vi "Shooter Speed Control.vi"(2 "Use Speed Control":bool=TRUE, 3 "Desired\nShooter\nSpeed":dbl) -> (1 "up to speed":bool)   [LabVIEW 2013]
panel:
  in  "counts/rev":dbl=240.0
  out "Wheel Speed R/sec":dbl=2.0076839341392278e-147 format="%#_4g"
  out "Count":i32=1335982
  in  "Reset Counter":bool
  in  "Speed avg. #":dbl=6.0
  in  "Gain":dbl=0.2
  in  "Allowable\nSpeed Error":dbl=2.0
  in  "Bias":dbl=99.0
  out "speed error":cluster{dbl, dbl}(graph)={-2.4092207209670736e-147, 0.017}
  # ".2"
  # "6"
  # "99"
  # "calibrate for \n50 rps with loop\ndisabled"
  # "240/360 depending\non which encoder\n\n81 on RPC test setup"
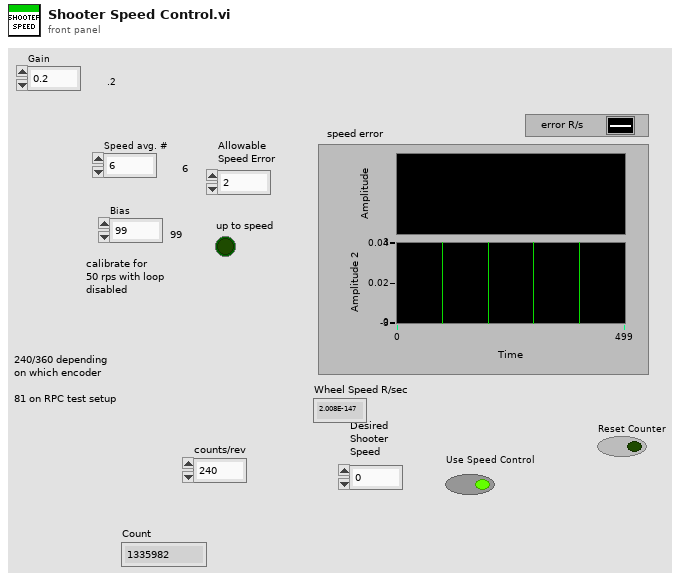
[diagram p1: front panel]
types:
  T1 = typedef "WPI_CounterDevRef.ctl" = cluster{"DevStatus":errorcluster, "CntIndex":T2}
  T2 = typedef "FPGA_CounterCtrSystemIndex.ctl" = enum8{"Ctr 0", "Ctr 1", "Ctr 2", "Ctr 3", "Ctr 4", "Ctr 5", "Ctr 6", "Ctr 7", "Invalid"}
  T3 = typedef "WPI_MotorControlDeviceRef.ctl" = cluster{"DeviceStatus":errorcluster, "Type":enum16{"PWM", "CAN"}, "PWM":cluster{"Digital Module":T4, "PWM Channel":T5, "DeadBand":T6}, "CAN":cluster{"Device Number":u8, "Control Mode":T7, "Semaphore":T8, "Max Vout":dbl}, "Invert":bool, "TransformRef":T9, "InvTransformRef":T9}
  T4 = typedef "FPGA_TypedefDigitalModule.ctl" = enum16{"Digital Module 1", "Digital Module 2"}
  T5 = typedef "FPGA_DIOPWMChannel.ctl" = enum8{"PWM 1", "PWM 2", "PWM 3", "PWM 4", "PWM 5", "PWM 6", "PWM 7", "PWM 8", "PWM 9", "PWM 10", "Invalid"}
  T6 = typedef "WPI_PWMDeadband.ctl" = cluster{"Name":string, "maxPositivePwm":i32, "minPositivePwm":i32, "centerPwm":i32, "maxNegativePwm":i32, "minNegativePwm":i32, "angularRange":u16}
  T7 = typedef "WPI_CANJaguar_ControlMode.ctl" = enum8{"Percent VBus", "Current", "Speed", "Position", "Voltage"}
  T8 = typedef "Semaphore RefNum" = refnum<k1>
  T9 = typedef "WPI_PWMTransform_ConPane.ctl" = refnum<vi>
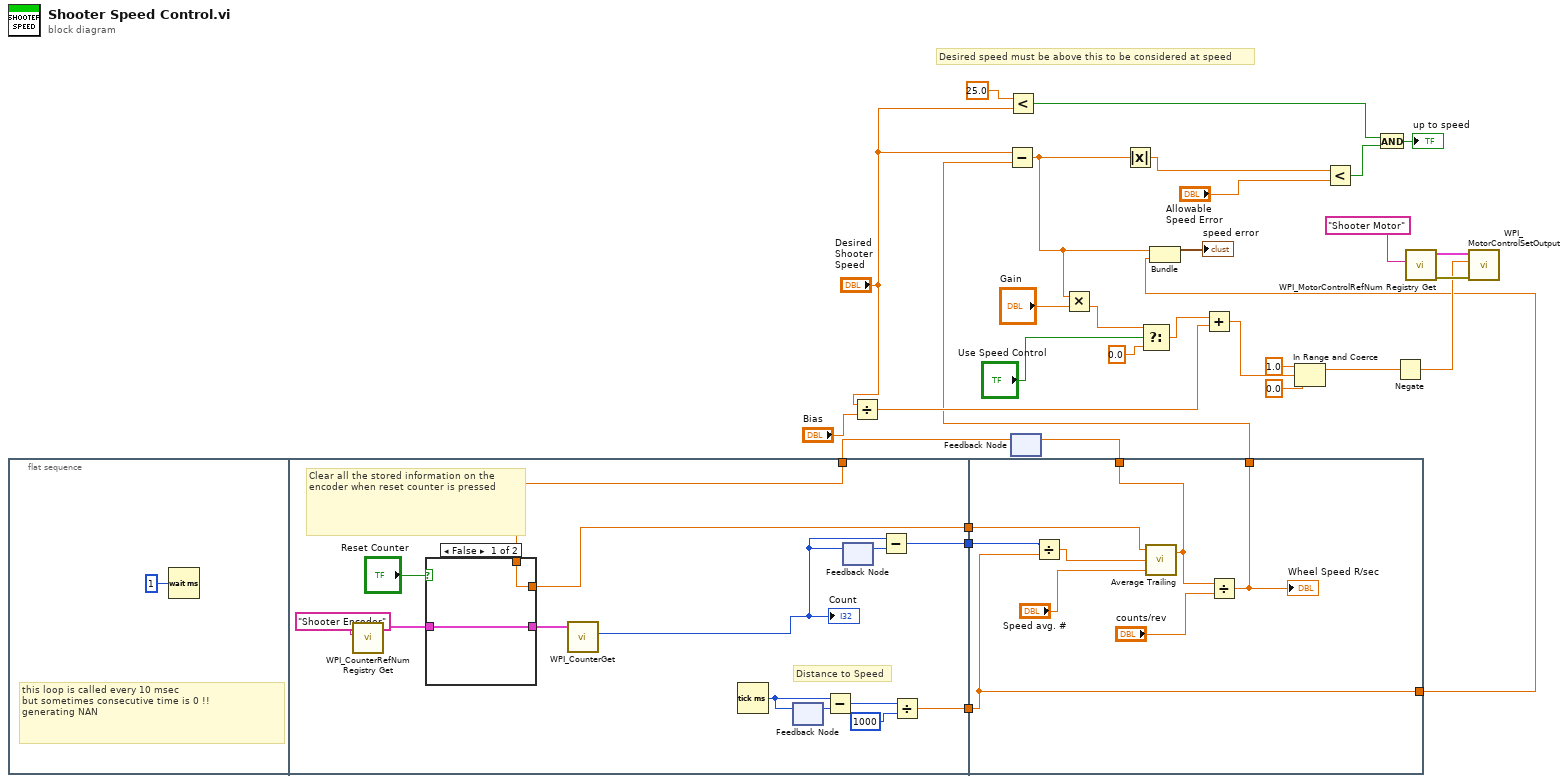
[diagram p0: block diagram]
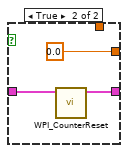
[diagram p2: hidden frame]
diagram:
  # "Desired speed must be above this to be considered at speed"
  n1 = flat-sequence {
    tunnel: [w36] -> w9
    tunnel: [w35] -> w8
    tunnel: [w34] -> w7
    tunnel: w1 -> [w33]
    tunnel: w9 -> [w56]
    tunnel: w8 -> [w54]
    tunnel: w7 -> [w55]
    tunnel: [w54] -> w6
    tunnel: [w53] -> w5
    tunnel: [w52] -> w2
    frame #0 {
      # "this loop is called every 10 msec\nbut sometimes consecutive time is 0 !!\ngenerating NAN"
      n2 = Wait (ms)(milliseconds to wait=u32 1) -> ()  [unwired: 1 out]
    }
    frame #1 {
      # "Distance to Speed"
      # "Clear all the stored information on the encoder when reset counter is pressed"
      n3 = call <vilib>:"WPI_CounterRefNum Registry Get.vi"("refnum name"="Shooter Encoder") -> ("CounterDevRef"=w41:T1)  [unwired: 9 in, 1 out]
      n4 = case shown="False" "Reset Counter" {
        tunnel: w41 -> [w48 w50]
        tunnel: [w48 w49] -> w38
        tunnel: w33 -> [w47 _]
        tunnel: [w47 0.0 ("Output")] -> w34
        frame False {
        }
        frame True {
          n5 = call <vilib>:"WPI_CounterReset.vi"("CounterDevRef in"=w50) -> ("CounterDevRef out"=w49:T1)  [unwired: 9 in, 1 out]
        }
      }
      n6 = call <vilib>:"WPI_CounterGet.vi"("CounterDevRef in"=w38) -> ("Value"=w37:i32)  [unwired: 5 in, 5 out]
      "Count" <- w37
      n7 = Tick Count (ms)() -> (millisecond timer value=w42:u32)
      n8 = feedback #1() -> (w43:u32)  [unwired: 1 in]
      n9 = feedback-in #1(w42) -> ()
      n10 = Subtract(x=w42, y=w43) -> (x-y=w45:u32)
      n11 = feedback #2() -> (w46:i32)  [unwired: 1 in]
      n12 = feedback-in #2(w37) -> ()
      n13 = Subtract(x=w37, y=w46) -> (x-y=w36:i32)
      n14 = Divide(x=w45, y=u32 1000) -> (x/y=w35:dbl)
    }
    frame #2 {
      n15 = Divide(x=w56, y=w54) -> (x/y=w57:dbl)
      n16 = call "Average Trailing.vi"("averg #"="Speed avg. #", "Input"=w57, "Previous\nValue"=w55) -> ("Output"=w52:dbl)  [unwired: 1 in]
      n17 = Divide(x=w52, y="counts/rev") -> (x/y=w53:dbl)
      "Wheel Speed R/sec" <- w53
    }
  }
  n18 = Divide(x="Desired\nShooter\nSpeed", y="Bias") -> (x/y=w24:dbl)
  n19 = Subtract(x="Desired\nShooter\nSpeed", y=w5) -> (x-y=w4:dbl)
  n20 = Less?(x=25.0, y="Desired\nShooter\nSpeed") -> (x < y?=w15:bool)
  n21 = feedback #3() -> (w1:dbl)  [unwired: 1 in]
  n22 = feedback-in #3(w2) -> ()
  n23 = Multiply(x=w4, y="Gain") -> (x*y=w13:dbl)
  n24 = Absolute Value(x=w4) -> (abs(x)=w26:dbl)
  n25 = Select(t=w13, s="Use Speed Control", f=0.0) -> (s? t:f=w18:dbl)
  n26 = Bundle(w4, w6) -> (→"speed error":cluster{dbl, dbl})  [unwired: 1 in]
  n27 = Add(x=w18, y=w24) -> (x+y=w22:dbl)
  n28 = In Range and Coerce(upper limit=1.0, x=w22, lower limit=0.0) -> (coerced(x)=w12:dbl)  [unwired: 1 out]
  n29 = Less?(x=w26, y="Allowable\nSpeed Error") -> (x < y?=w28:bool)
  n30 = And(x=w15, y=w28) -> (x .and. y?=→"up to speed":bool)
  n31 = Negate(x=w12) -> (-x=w11:dbl)
  n32 = call <vilib>:"WPI_MotorControlRefNum Registry Get.vi"("refnum name"="Shooter Motor") -> ("error out"=w30:errorcluster, "MotorControlDevRef"=w31:T3)  [unwired: 9 in]
  n33 = call <vilib>:"WPI_MotorControlSetOutput.vi"("error in (no error)"=w30, "Output"=w11, "MotorControlDevRef"=w31) -> ()  [unwired: 6 in, 3 out]
